vi "unused_shift_singleDirection.vi"(6 "direction":T1, 8 "error in (no error)":errorcluster, 10 "delta[pixel]":i32, 11 "GObject in":refnum<class "Generic.lvclass">) -> (0 "error out":errorcluster, 3 "GObject out":refnum<class "Generic.lvclass">)   [LabVIEW 2023]
uses:
  Generic.lvclass
  Ctrls/direction.ctl
  Generic.lvclass/Generic.ctl
  TLC_Scripto.lvlib
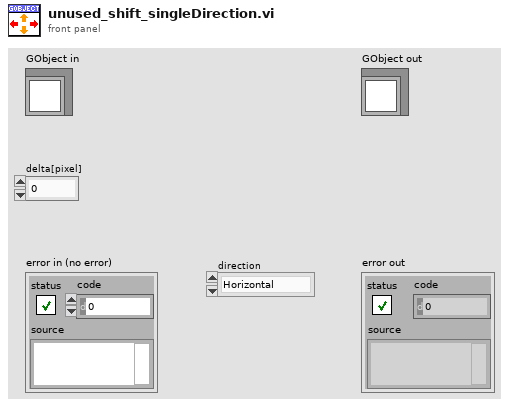
[diagram p1: front panel]
types:
  T1 = typedef "TLC_Scripto.lvlib/direction.ctl" = enum16{"Horizontal", "Vertical"}
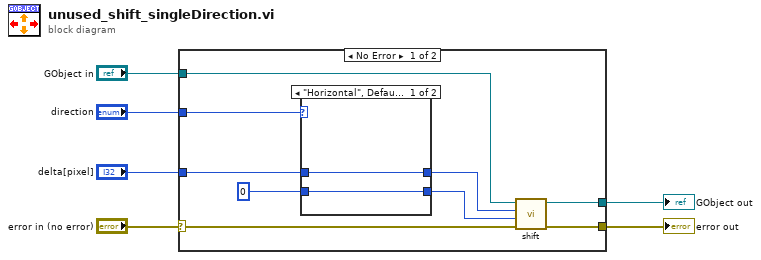
[diagram p0: block diagram]
diagram:
  n1 = case shown="No Error" "error in (no error)" {
    selector: "error in (no error)" -> [w15 w21]
    tunnel: [w14 w21] -> w5
    tunnel: [w13 w20] -> w3
    tunnel: "GObject in" -> [w12 w20]
    tunnel: "delta[pixel]" -> [w7 _]
    tunnel: "direction" -> [w11 _]
    frame No Error {
      n2 = case shown="\"Horizontal\", Default" w11 {
        tunnel: 0 ("deltaX_[pixel]") -> [w17 w19]
        tunnel: [w17 w18] -> w9
        tunnel: [w16 w19] -> w8
        tunnel: w7 -> [w16 w18]
        frame "Horizontal", Default {
        }
        frame "Vertical" {
        }
      }
      n3 = call-dynamic "shift.vi"("error in (no error)"=w15, "deltaY[pixel]"=w9, "deltaX_[pixel]"=w8, "GObject in"=w12) -> ("error out"=w14:errorcluster, "GObject out"=w13:refnum<class "Generic.lvclass">)  [unwired: 6 in]
    }
    frame Error {
    }
  }
  "error out" <- w5
  "GObject out" <- w3
